vi "Get Data.vi"(8 "error in":errorcluster, 11 "SDO Transfer in":refnum<class "SDO Transfer.lvclass">) -> (0 "error out":errorcluster, 2 "Data":u8[](array[numeric]) format="%02x", 3 "SDO Transfer out":refnum<class "SDO Transfer.lvclass">)   [LabVIEW 2020, in "CANopen.lvlib" / "SDO Manager.lvlib" / "SDO Transfer.lvclass"]
uses:
  SDO Transfer.lvclass
  SDO Transfer.lvclass/SDO Transfer.ctl
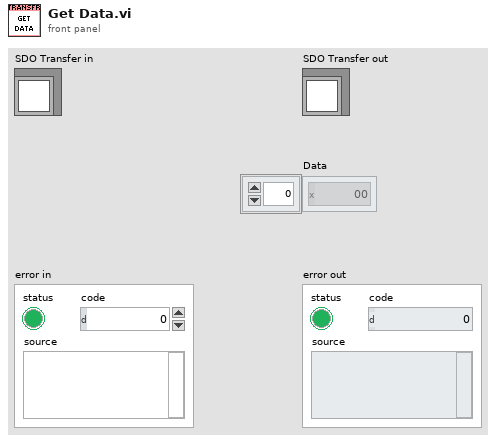
[diagram p1: front panel]
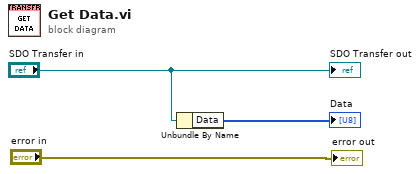
[diagram p0: block diagram]
diagram:
  n1 = Unbundle By Name("SDO Transfer in") -> ("Data"=→"Data":u8[])
  "SDO Transfer out" <- "SDO Transfer in"
  "error out" <- "error in"
